vi "LM_HslCommunication Demo.vi"() -> ()   [LabVIEW 2018]
uses:
  Class/Seimens.lvclass
  <vilib>/Utility/error.llb/DialogType.ctl
  Class/Public/Read/SeimensS7Net_ReadUInt16[].vi
  Class/Public/Write/SeimensS7Net_WriteInt16[].vi
panel:
  in  "error in (no error)":errorcluster caption="错误输入（无错误）"
  in  "WriteAddress":string="DB2.0"
  in  "WriteValues":u16[](array[numeric])
  out "ReadArray":u16[](array[numeric])
  in  "Write":bool
  out "error out":errorcluster caption="错误输出"
  in  "ReadLength":u16=1
  in  "ReadAddress":string="DB2.0"
  in  "停止":bool
  # "Read"
  # "Write"
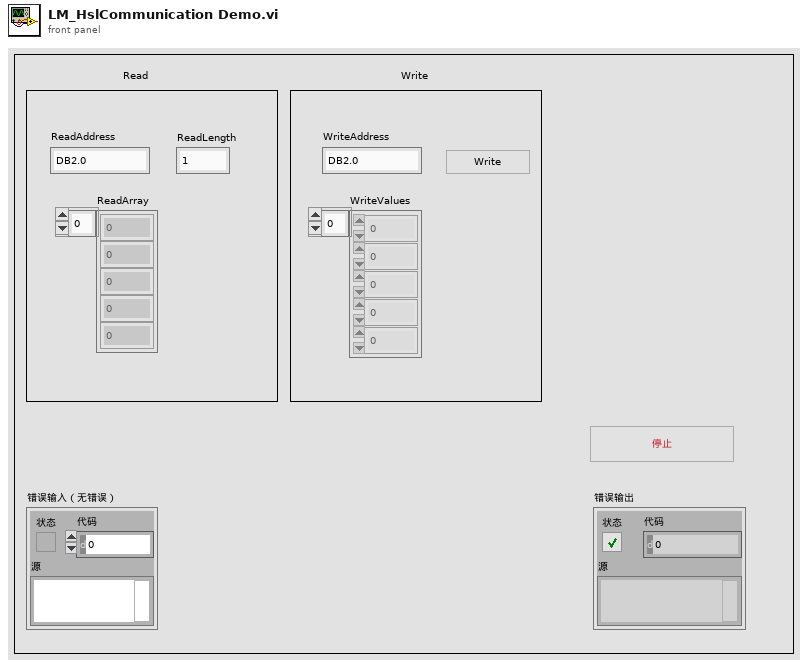
[diagram p1: front panel]
types:
  T1 = typedef "DialogType.ctl" = u16
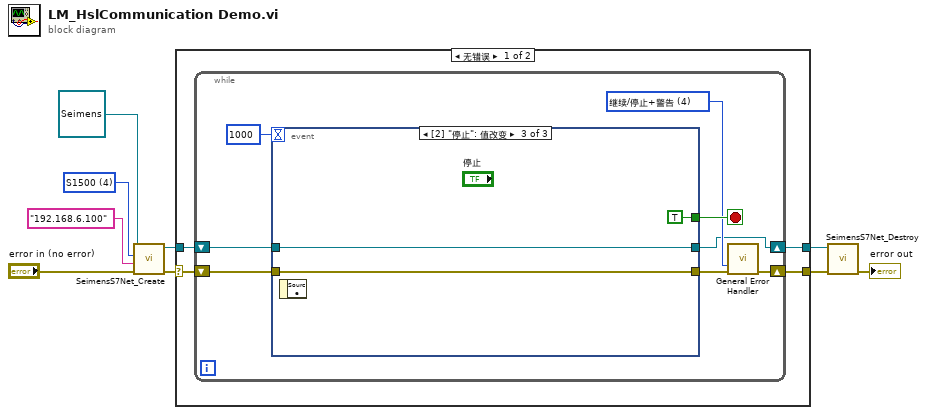
[diagram p0: block diagram]
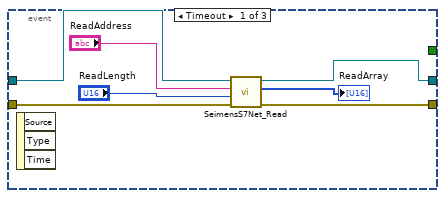
[diagram p2: hidden frame]
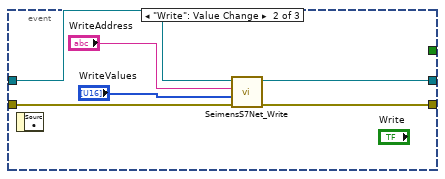
[diagram p3: hidden frame]
diagram:
  w4 = 4 items=["S1200"=1, "S300"=2, "S400"=3, "S1500"=4, "S200Smart"=5, "S200"=6] ("siemens")
  n1 = call "SeimensS7Net_Create.vi"("error in (no error)"="error in (no error)", "ipAddress"="192.168.6.100", "siemens"=w4, "Seimens 输入"=refnum<class "Seimens.lvclass"> refnum) -> ("error out"=w9:errorcluster, "Seimens 输出"=w8:refnum<class "Seimens.lvclass">)  [unwired: 6 in]
  n2 = case shown="无错误" w9 {
    selector: w9 -> [w12 w39]
    tunnel: w8 -> [w13 w38]
    tunnel: [w11 w38] -> w7
    tunnel: [w10 w39] -> w6
    frame No Error {
      n3 = while {
        shift-right: [w14] -> w11
        shift-left: w13 -> [w19]
        shift-right: [w16] -> w10
        shift-left: w12 -> [w18]
        stop <- w21 stop-if-true
        w15 = T1 4 items=["无对话框", "确定信息", "继续或停止信息", "确定信息＋警告", "继续/停止+警告"] ("type of dialog (OK msg:1)")
        n4 = event shown="[2] \"停止\": 值改变" {
          selector: _ -> [_ _ _]
          dyn-events: _ -> [_ _ _]
          timeout: 1000 -> [_ _ _]
          tunnel: [_ _ TRUE] -> w21
          tunnel: w19 -> [w28 w34 w36]
          tunnel: [w27 w31 w36] -> w14
          tunnel: w18 -> [w24 w33 w35]
          tunnel: [w23 w32 w35] -> w17
          event Timeout {
            n5 = event-data() -> ()  [unwired: 1 in, 3 out]
            n6 = call-poly "SeimensS7Net_Read.vi"("error in (no error)"=w24, "length"="ReadLength", "address"="ReadAddress", "Seimens 输入"=w28) -> ("error out"=w23:errorcluster, "ReadArray"=→"ReadArray":u16[], "Seimens 输出"=w27:refnum<class "Seimens.lvclass">)  [unwired: 5 in]
          }
          event "Write": Value Change {
            n7 = event-data() -> ()  [unwired: 1 in, 1 out]
            n8 = call-poly "SeimensS7Net_Write.vi"("error in (no error)"=w33, "values"="WriteValues", "address"="WriteAddress", "Seimens 输入"=w34) -> ("error out"=w32:errorcluster, "Seimens 输出"=w31:refnum<class "Seimens.lvclass">)  [unwired: 5 in, 1 out]
          }
          event "停止": Value Change {
            n9 = event-data() -> ()  [unwired: 1 in, 1 out]
          }
        }
        n10 = call <vilib>:"General Error Handler.vi"("type of dialog (OK msg:1)"=w15, "error in (no error)"=w17) -> ("error out"=w16:errorcluster)  [unwired: 9 in, 4 out]
      }
    }
    frame Error {
    }
  }
  n11 = call "SeimensS7Net_Destroy.vi"("error in (no error)"=w6, "Seimens 输入"=w7) -> ("error out"=→"error out":errorcluster)  [unwired: 9 in]
